vi "last 20 array elements.vi"(9 "number to be inserted at end":dbl, 10 "input array":dbl[](array[numeric])) -> (2 "output array":dbl[](array[numeric]))   [LabVIEW 2009, in "Varian.lvlib"]
uses:
  Varian.lvlib
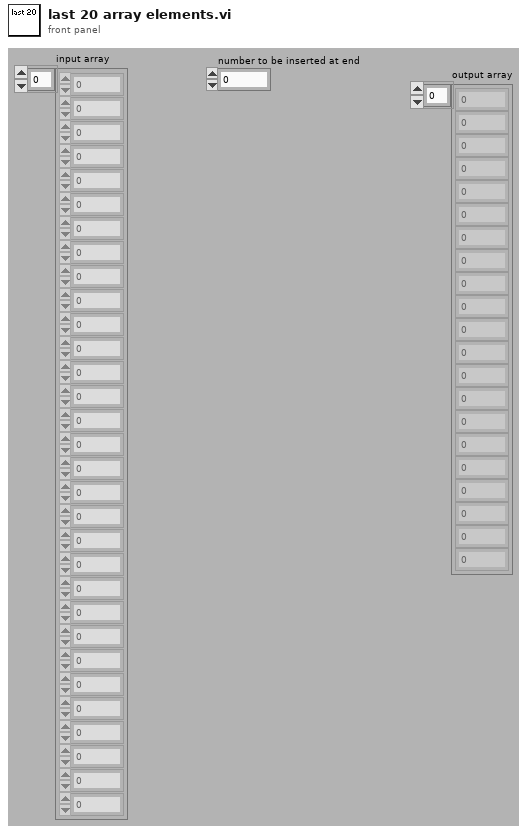
[diagram p1: front panel]
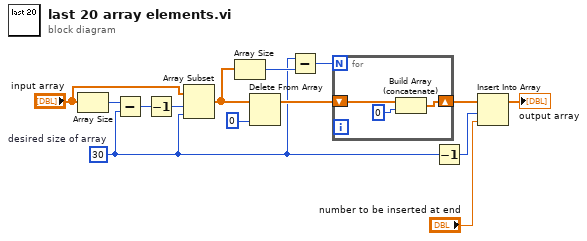
[diagram p0: block diagram]
diagram:
  w3 = 30  # desired size of array
  n1 = Array Size(array="input array") -> (size(s)=w4:i32)
  n2 = Subtract(x=w4, y=w3) -> (x-y=w2:i32)
  n3 = Decrement(x=w2) -> (x-1=w1:i32)
  n4 = Array Subset(array="input array", index=w1, length=w3) -> (w6:dbl[])
  n5 = Array Size(array=w6) -> (size(s)=w11:i32)
  n6 = Delete From Array(array=w6, index=0) -> (array with subset deleted=w10:dbl[])  [unwired: 1 in, 1 out]
  n7 = Subtract(x=w3, y=w11) -> (x-y=w7:i32)
  n8 = for {
    N: w7 -> [_]
    shift-right: [w15] -> w9
    shift-left: w10 -> [w17]
    n9 = Build Array (concatenate)(w17, 0) -> (w15:dbl[])
  }
  n10 = Decrement(x=w3) -> (x-1=w8:i32)
  n11 = Insert Into Array(array=w9, index=w8, new element="number to be inserted at end") -> (→"output array":dbl[])
